vi "Load Display Settings from File.vi"(0 "Display State In":T1 {"ROI"."Contours"."Type" items=["No Selection", "Point", "Line", "Rectangle", "Oval", "Polygon", "Freehand Region", "Annulus", "Unused2", "Unused3", "Broken Line", "Freehand Line", "Rotated Rectangle"]}, 9 "Container State":T7, 11 "error in (no error)":errorcluster) -> (4 "Display State Out":T1 {"ROI"."Contours"."Type" items=["No Selection", "Point", "Line", "Rectangle", "Oval", "Polygon", "Freehand Region", "Annulus", "Unused2", "Unused3", "Broken Line", "Freehand Line", "Rotated Rectangle"]}, 15 "error out":errorcluster)   [LabVIEW 2009, in "POLARIS IMAQ Display.xctl"]
uses:
  POLARIS IMAQ Display.xctl
  <vilib>/_xctls/Container State.ctl
  State.ctl
  IMAQdx Cam/IMAQdx Cam.lvclass
  Properties/ImageSource.ctl
  <vilib>/vision/Image Controls.llb/IMAQ Image.ctl
  DisplaySettings.ctl
  Named ROI.ctl
  Analyze Classes/Analyze BaseClass/Analyze BaseClass.lvclass
  <vilib>/_xctls/XControlSupport.lvlib
panel:
  # "Add Controls & Indicators that form the parameters of the method here. Hook them to the connector pane. Do not delete the controls & indicators that are already hooked to the connector pane.\n \nTo setup the parameters  for this method, right click on this item in the Project Tree & select \"Configure Method...\"."
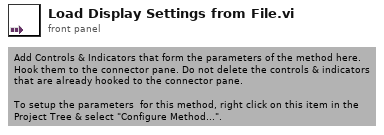
[diagram p1: front panel]
types:
  T1 = typedef "POLARIS IMAQ Display.xctl/State.ctl" = cluster{"ImageSource":T2, "IMAQdx Cam":refnum<class "IMAQdx Cam.lvclass">, "WorkDir":path, "Image Name Prefix":string, "ROI":T3, "BG Image":T4, "Display Image":T4, "Display settings":T5, "Mask image":T4, "ConfigDir":path, "Display ref":refnum<vi>, "Saved ROIs":T6[], "Selected ROI":string, "Analyze Objects":refnum<class "Analyze BaseClass.lvclass">[], "Analysis Params":variant, "Analysis Results":variant, "Overlays?":bool[], "UPaleteTeiler Ref":refnum<vi>, "Ref Palette type":refnum<vi>, "Time in Filename?":bool, "Save Report?":bool}
  T2 = typedef "POLARIS IMAQ Display.xctl/ImageSource.ctl" = enum16{"Camera", "File"}
  T3 = typedef "ROI Descriptor" = cluster{"Global Rectangle":i32[], "Contours":cluster{"ID":enum32{"External", "Internal"}, "Type":u32, "Coordinates":i32[]}[]}
  T4 = typedef "IMAQ Image.ctl" = refnum<image>
  T5 = typedef "POLARIS IMAQ Display.xctl/DisplaySettings.ctl" = cluster{"Min. Thresh.":sgl, "X":dbl, "Y":dbl, "ShowLineout":bool, "ScaleParts":i32, "ShowLegende":bool, "Target Cross":bool, "Centroid Cross":bool, "Target color":u32, "Centroid color":u32, "calibr. mm/px":sgl}
  T6 = typedef "POLARIS IMAQ Display.xctl/Named ROI.ctl" = cluster{"ROI":cluster{"Global Rectangle":i32[], "Contours":cluster{"Contour Type":u32, "ROI Type":u32, "Points":i32[]}[]}, "Name":string}
  T7 = typedef "XControlSupport.lvlib/Container State.ctl" = cluster{"Indicator?":bool, "Run Mode?":bool, " Refnum":refnum<vi>}
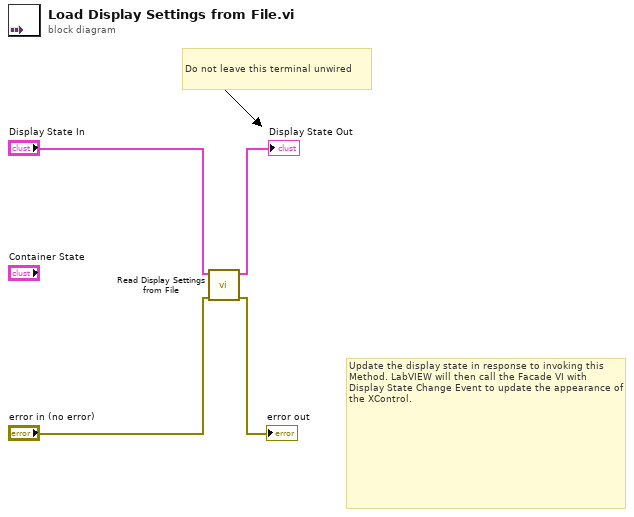
[diagram p0: block diagram]
diagram:
  # "Do not leave this terminal unwired"
  # "Update the display state in response to invoking this Method. LabVIEW will then call the Facade VI with Display State Change Event to update the appearance of the XControl."
  n1 = call "Read Display Settings from File.vi"("error in (no error)"="error in (no error)", "State in"="Display State In") -> ("error out"=→"error out":errorcluster, "State out"=→"Display State Out":T1)  [unwired: 8 in]
